vi "06b-arrays.vi"() -> ()   [LabVIEW 2018, in "LV-0mq-Julia_roundtrip-lib.lvlib"]
uses:
  LV-0mq-Julia_roundtrip-lib.lvlib
  Server or client state.ctl
  detailed error info.ctl
  StackFrame.ctl
  Commands.ctl
  0d29fc62-3d1d-4713-a954-9c9e873b3633.vi
  aea790a6-a42b-4eb0-905f-734239196901.vi
  <vilib>/Analysis/7linalg.llb/Solve Linear Equations (single right hand).vi
  72a46192-383e-4ee5-9465-71670922b82a.vi
  ef5408d4-6538-41d1-b296-fda05a71e4b0.vi
  446b7249-21ad-448f-9866-a149977bd6ec.vi
  e4efb182-1b04-4d49-96a3-1defebd055ea.vi
  0d29fc62-3d1d-4713-a954-9c9e873b3633.vi/8ee49078-a04b-40cf-aceb-de90d52f19ef.vi
  aea790a6-a42b-4eb0-905f-734239196901.vi/353007a7-a356-474a-8eac-0d4386ef6058.vi
  <vilib>/Analysis/baseanly.llb/Solve Linear Equations By Cholesky.vi
  <vilib>/Analysis/baseanly.llb/Real Matrix to Compact Array.vi
  <vilib>/Analysis/baseanly.llb/Real Compact Tri-Matrix Linear Eqs.vi
  72a46192-383e-4ee5-9465-71670922b82a.vi/ea2ca31c-a649-493c-8d06-3a8000b732b1.vi
  ef5408d4-6538-41d1-b296-fda05a71e4b0.vi/365813fc-9c19-4b31-a490-477dd90e6dd4.vi
  446b7249-21ad-448f-9866-a149977bd6ec.vi/13d8bec3-26a9-4f1a-9c06-75e8e16d8110.vi
  e4efb182-1b04-4d49-96a3-1defebd055ea.vi/2d8ce8de-4b8b-497d-8f47-069ef3484173.vi
  e4efb182-1b04-4d49-96a3-1defebd055ea.vi/ce0a9de1-ea0e-471e-bc56-afcb036c643e.vi
  72a46192-383e-4ee5-9465-71670922b82a.vi/ea2ca31c-a649-493c-8d06-3a8000b732b1.vi/4cda02a8-52b1-4797-9517-7736628fdc16.vi
  ef5408d4-6538-41d1-b296-fda05a71e4b0.vi/365813fc-9c19-4b31-a490-477dd90e6dd4.vi/c1bf83d8-4e50-4008-8373-782bae7d23a9.vi
  446b7249-21ad-448f-9866-a149977bd6ec.vi/13d8bec3-26a9-4f1a-9c06-75e8e16d8110.vi/92273e5d-2cd6-461b-92a5-92ae252801d6.vi
  446b7249-21ad-448f-9866-a149977bd6ec.vi/13d8bec3-26a9-4f1a-9c06-75e8e16d8110.vi/e0261a75-2649-47ad-afbf-694dd59d57de.vi
  446b7249-21ad-448f-9866-a149977bd6ec.vi/13d8bec3-26a9-4f1a-9c06-75e8e16d8110.vi/e4df3bbc-3abc-4d2a-94de-58760ccb0cd8.vi
  e4efb182-1b04-4d49-96a3-1defebd055ea.vi/2d8ce8de-4b8b-497d-8f47-069ef3484173.vi/ef05d8d3-eacc-4a0c-93e4-778c0cfb98e9.vi
  e4efb182-1b04-4d49-96a3-1defebd055ea.vi/2d8ce8de-4b8b-497d-8f47-069ef3484173.vi/14059dc4-69a7-4969-bd3d-bae21b85096e.vi
  72a46192-383e-4ee5-9465-71670922b82a.vi/ea2ca31c-a649-493c-8d06-3a8000b732b1.vi/4cda02a8-52b1-4797-9517-7736628fdc16.vi/f6bd3a2a-1504-4020-af9c-daf7937f7973.vi
  ef5408d4-6538-41d1-b296-fda05a71e4b0.vi/365813fc-9c19-4b31-a490-477dd90e6dd4.vi/c1bf83d8-4e50-4008-8373-782bae7d23a9.vi/fa26639b-d519-4ace-9d6a-dd3a988d1d0b.vi
  e4efb182-1b04-4d49-96a3-1defebd055ea.vi/2d8ce8de-4b8b-497d-8f47-069ef3484173.vi/ef05d8d3-eacc-4a0c-93e4-778c0cfb98e9.vi/892bfb83-c346-4c76-9c4d-d6d5bca15b91.vi
  jl-scripts path.vi
  <vilib>/Analysis/7linalg.llb/Solve Linear Eqs (General).vi
  <vilib>/Analysis/7linalg.llb/Solve Linear Eqs (Gen, single right hand).vi
  check ID validity.vi
  bindata_descr to JSON.vi
  check cluster field names.vi
  concat JSON.vi
  build request.vi
  Parse server response.vi
  log jl exceptions.vi
  <vilib>/Utility/error.llb/Error Cluster From Error Code.vi
  <vilib>/Analysis/NI_AALPro.lvlib
panel:
  out "max difference":dbl format="%#_3e"
  in  "arr size N":u16=4
  out "Solution Vector":dbl[](array[numeric]) format="%.2f"
  out "Known Vector":dbl[](array[numeric])=[22.0, 14.0, 18.0]
  out "Input Matrix (NxN)":dbl[][](array[numeric])=[[1.0, 0.0, 5.0], [4.0, 2.0, 1.0], [2.0, 2.0, 3.0]]
  in  "next":bool
  out "detailed error info":T1
  out "current error":errorcluster
  out "final error":errorcluster
  out "short err code":u8
  in  "stop":bool
  out "ZMQ timeout":bool
  out "Julia script file path":path
  out "temporary script path":path
  out "Jl Server state":T3
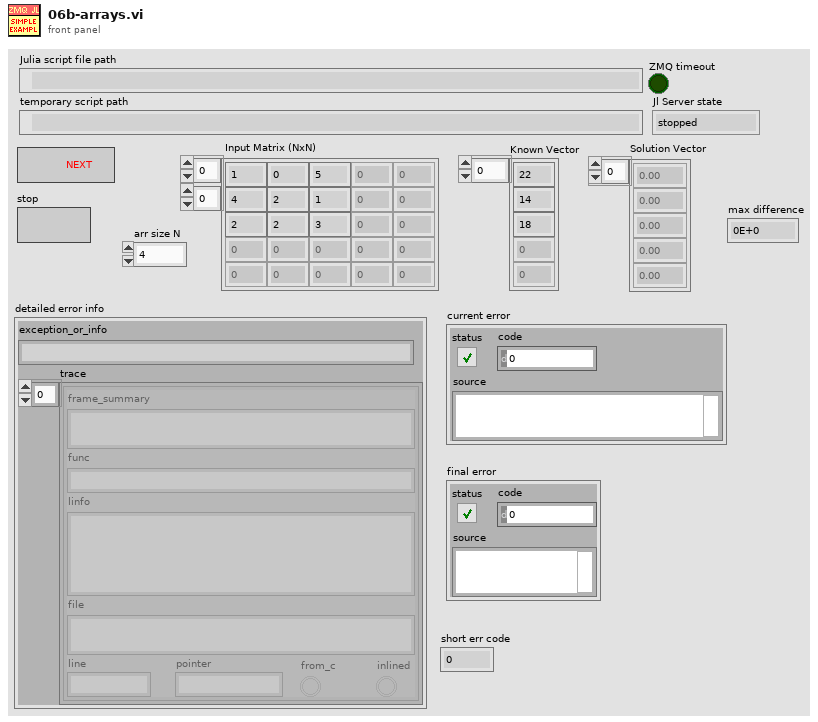
[diagram p1: front panel]
types:
  T1 = typedef "LV-0mq-Julia_roundtrip-lib.lvlib/detailed error info.ctl" = cluster{"exception_or_info":string, "trace":T2[]}
  T2 = typedef "LV-0mq-Julia_roundtrip-lib.lvlib/StackFrame.ctl" = cluster{"frame_summary":string, "func":string, "linfo":string, "file":string, "line":i32, "pointer":u64, "from_c":bool, "inlined":bool}
  T3 = typedef "LV-0mq-Julia_roundtrip-lib.lvlib/Server or client state.ctl" = enum16{"stopped", "running", "unknown"}
  T4 = typedef "LV-0mq-Julia_roundtrip-lib.lvlib/Commands.ctl" = enum16{"Start Jl-server & Init LV-client", "Send request & Get response ", "Stop Jl-server & Cleanup LV-client", "Cleanup LV-client", "Start Jl-server", "Stop Jl-server", "Init LV-Client", "Cleanup LV-Client", "(not allowed)", "Set LV Client state", "Set Jl Server state", "set ZMQ timeout", "read ZMQ timeout", "read-out state"}
  T5 = typedef "LV-0mq-Julia_roundtrip-lib.lvlib/Bindata&description.ctl" = cluster{"bindata_descr":T6[], "bindata":u8[]}
  T6 = typedef "LV-0mq-Julia_roundtrip-lib.lvlib/Bindata description.ctl" = cluster{"nofbytes":i32, "numtype":string, "start":i32, "arrdims":i32[], "kwarg_name":string, "category":string}
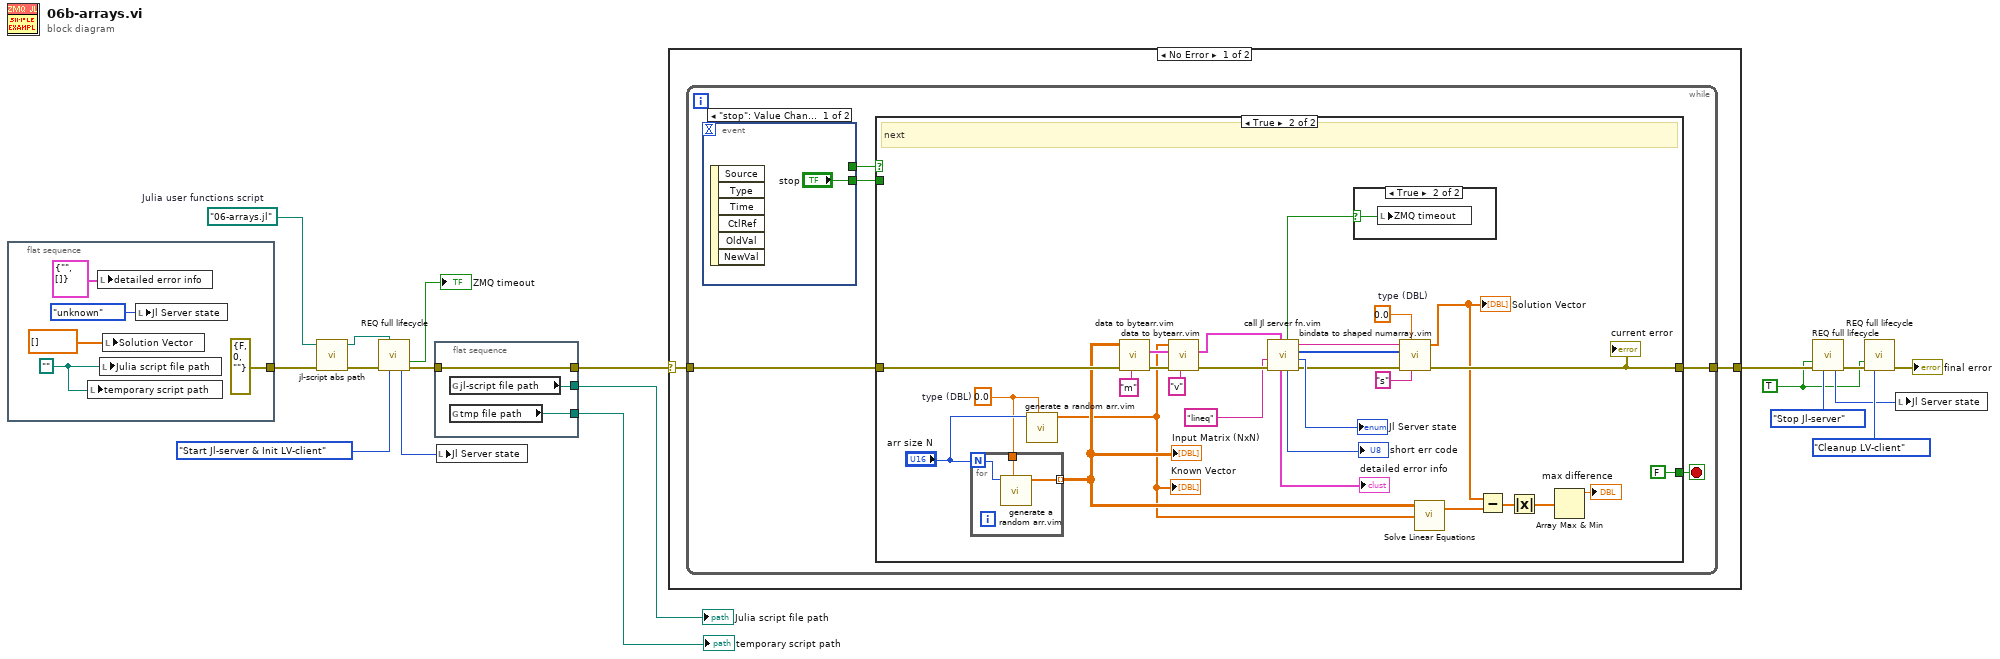
[diagram p0: block diagram]
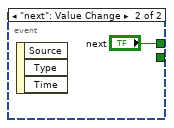
[diagram p2: hidden frame]
diagram:
  w4 = path "06-arrays.jl"  # Julia user functions script
  w1 = TRUE ("Force command")
  n1 = flat-sequence {
    tunnel: [errorcluster {"status"=FALSE, "code"=0, "source"=""} ("error in (no error)")] -> w2
    frame #0 {
      w19 = path ""
      n2 = local write "temporary script path"(w19) -> ()
      n3 = local write "detailed error info"(T1 {"exception_or_info"="", "trace"=[]} ("detailed error info")) -> ()
      n4 = local write "Julia script file path"(w19) -> ()
      n5 = local write "Solution Vector"(dbl[] [] ("Server response")) -> ()
      n6 = local write "Jl Server state"(Server_or_client_state."unknown" ("Jl Server state out")) -> ()
    }
  }
  n7 = call "jl-script abs path.vi"("error in (no error)"=w2, "Julia user functions script"=w4) -> ("error out"=w5:errorcluster, "script abs path"=w6:path)  [unwired: 8 in]
  n8 = call "REQ full lifecycle.vi"("Julia user functions script"=w6, "error in"=w5, "command"=Commands."Start Jl-server & Init LV-client") -> ("timeout?"=→"ZMQ timeout":bool, "Jl Server state out"=w8:T3, "error out"=w7:errorcluster)  [unwired: 6 in, 4 out]
  n9 = flat-sequence {
    tunnel: [w26] -> w13
    tunnel: w7 -> [w26]
    tunnel: [w25] -> w11
    tunnel: [w24] -> w12
    frame #0 {
      n10 = global read "jl-scripts path.vi" "jl-script file path"() -> (w25:path)
      n11 = global read "jl-scripts path.vi" "tmp file path"() -> (w24:path)
    }
  }
  n12 = local write "Jl Server state"(w8) -> ()
  n13 = case shown="No Error" w13 {
    selector: w13 -> [w27 w70]
    tunnel: [w28 w70] -> w18
    frame No Error {
      n14 = while {
        tunnel: w27 -> [w32]
        tunnel: [w33] -> w28
        stop <- w30 stop-if-true
        n15 = event shown="[0] \"stop\": Value Change" {
          selector: _ -> [_ _]
          dyn-events: _ -> [_ _]
          timeout: _ -> [_ _]
          tunnel: [_ "next"] -> w31
          tunnel: ["stop" _] -> w29
          event "stop": Value Change {
            n16 = event-data() -> ()  [unwired: 1 in, 6 out]
          }
          event "next": Value Change {
            n17 = event-data() -> ()  [unwired: 1 in, 3 out]
          }
        }
        n18 = case shown="True" w31 {
          tunnel: [w37 w59] -> w33
          tunnel: w32 -> [w37 w62]
          tunnel: [w36 FALSE ("stop this VI only")] -> w30
          tunnel: w29 -> [w36 _]
          frame False {
            # "stop"
          }
          frame True {
            w55 = 0.0  # type (DBL)
            w58 = 0.0  # type (DBL)
            # "next"
            n19 = for {
              N: "arr size N" -> [w66]
              tunnel: [w68] -> w54 mode=indexing
              tunnel: w55 -> [w67]
              n20 = call "generate a random arr.vim"("type in"=w67, "arr size"=w66) -> ("float out"=w68:dbl[])  [unwired: 5 in, 4 out]
            }
            "Input Matrix (NxN)" <- w54
            n21 = call "generate a random arr.vim"("type in"=w55, "arr size"="arr size N") -> ("float out"=w53:dbl[])  [unwired: 5 in, 4 out]
            "Known Vector" <- w53
            n22 = call "data to bytearr.vim"("kwarg_name"="m", "error in (no error)"=w62, "data in"=w54) -> ("error out"=w64:errorcluster, "Bindata & descr out"=w63:T5)  [unwired: 6 in, 1 out]
            n23 = call "data to bytearr.vim"("kwarg_name"="v", "error in (no error)"=w64, "Bindata & descr in"=w63, "data in"=w53) -> ("error out"=w47:errorcluster, "Bindata & descr out"=w41:T5)  [unwired: 5 in, 1 out]
            n24 = call "call Jl server fn.vim"("Bindata & descr in"=w41, "error in (no error)"=w47, "fun2call"="lineq" ("Julia function name")) -> ("error out"=w42:errorcluster, "Jl Server state out"=→"Jl Server state":T3, "binary data received"=w38:u8[], "JSON received"=w39:string, "return code"=→"short err code":u8, "timeout?"=w40:bool, "detailed error info"=→"detailed error info":T1)  [unwired: 2 in]
            n25 = case shown="True" w40 {
              selector: w40 -> [_ w69]
              frame False {
              }
              frame True {
                n26 = local write "ZMQ timeout"(w69) -> ()
              }
            }
            n27 = call "bindata to shaped numarray.vim"("kwarg_name"="s", "data type"=w58, "error in (no error)"=w42, "binary data"=w38, "JSON in"=w39) -> ("error out"=w59:errorcluster, "numarray 1D"=w52:dbl[])  [unwired: 3 in, 2 out]
            "current error" <- w59
            "Solution Vector" <- w52
            n28 = call-poly <vilib>:"Solve Linear Equations.vi"("Known Vector"=w53, "Input Matrix"=w54) -> ("Solution Vector"=w51:dbl[])  [unwired: 1 in, 1 out]
            n29 = Subtract(x=w52, y=w51) -> (x-y=w50:dbl[])
            n30 = Absolute Value(x=w50) -> (abs(x)=w49:dbl[])
            n31 = Array Max & Min(array=w49) -> (max value=→"max difference":dbl)  [unwired: 3 out]
          }
        }
      }
    }
    frame Error {
    }
  }
  n32 = call "REQ full lifecycle.vi"("Force command"=w1, "error in"=w18, "command"=Commands."Stop Jl-server") -> ("Jl Server state out"=w10:T3, "error out"=w16:errorcluster)  [unwired: 6 in, 5 out]
  n33 = call "REQ full lifecycle.vi"("Force command"=w1, "error in"=w16, "command"=Commands."Cleanup LV-client") -> ("error out"=→"final error":errorcluster)  [unwired: 6 in, 6 out]
  n34 = local write "Jl Server state"(w10) -> ()
  "temporary script path" <- w12
  "Julia script file path" <- w11
